vi "brat robotic.vi"() -> ()   [LabVIEW 2018]
uses:
  <vilib>/picture/3D Picture Control/Object/Create Object (name).vi
  <vilib>/picture/3D Picture Control/NI_3D Picture Control.lvlib
panel:
  in  "Angle":sgl(knob) scale=0.0..10.0
  in  "Axis":cluster{"X":sgl, "Y":sgl, "Z":sgl}
  in  "Y":sgl(slide)=-0.010994764 scale=-0.7..0.7
  in  "X":sgl(slide)=0.0074074073 scale=-0.7..0.7
  in  "stop":bool
  out "3D Picture":refnum<vi>(3d-picture)
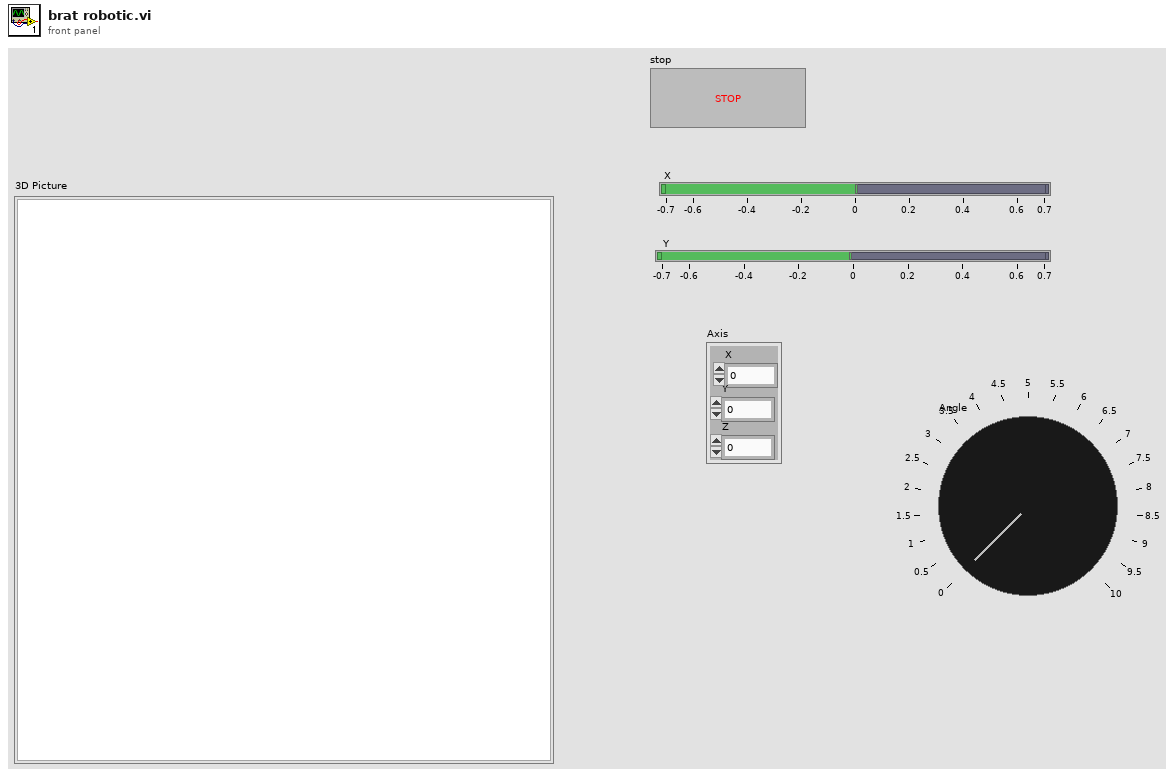
[diagram p1: front panel]
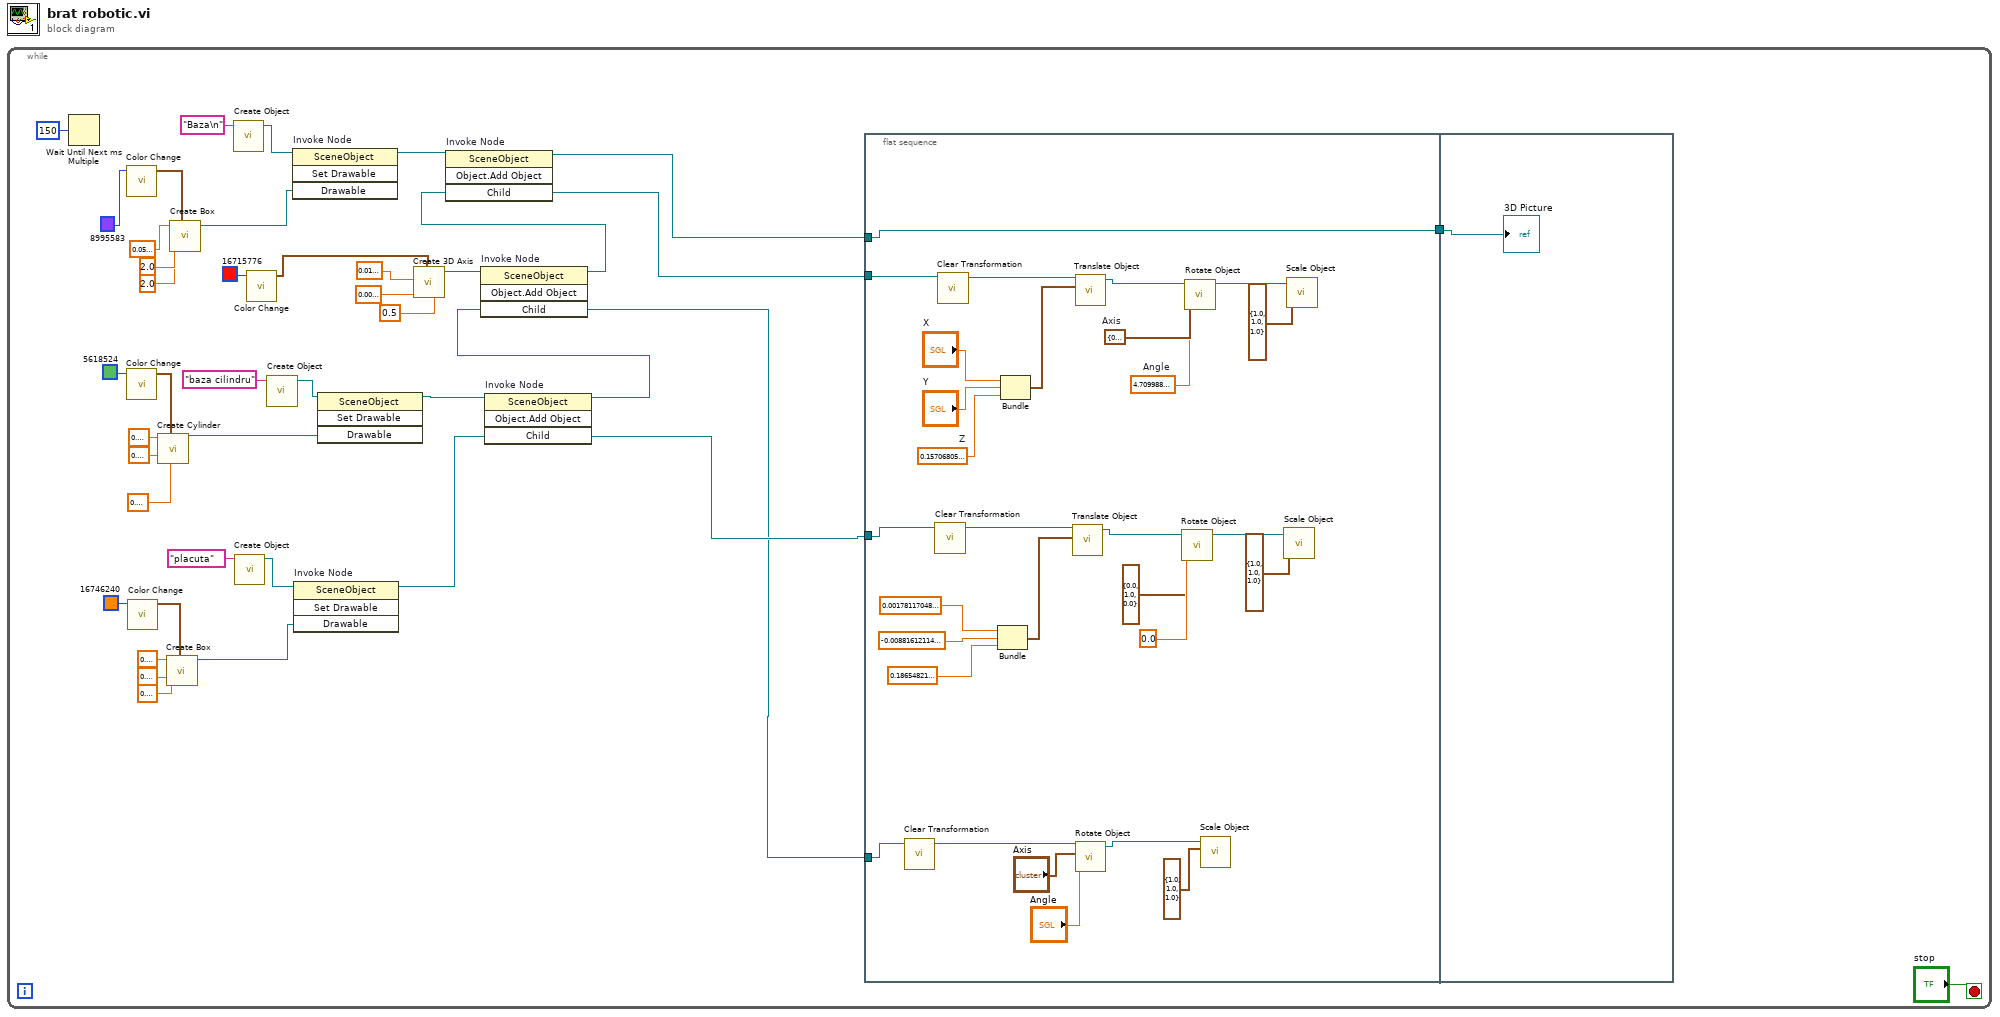
[diagram p0: block diagram]
diagram:
  n1 = while {
    stop <- "stop" stop-if-true
    n2 = Wait Until Next ms Multiple(millisecond multiple=u32 150) -> ()  [unwired: 1 out]
    n3 = call <vilib>:"Color Change.vi"("Color"=u32 8995583) -> ("RGBA"=w38:cluster{"R":sgl, "G":sgl, "B":sgl, "A":sgl})  [unwired: 10 in]
    n4 = call <vilib>:"Color Change.vi"("Color"=u32 5618524) -> ("RGBA"=w26:cluster{"R":sgl, "G":sgl, "B":sgl, "A":sgl})  [unwired: 10 in]
    n5 = call <vilib>:"Color Change.vi"("Color"=u32 16746240) -> ("RGBA"=w16:cluster{"R":sgl, "G":sgl, "B":sgl, "A":sgl})  [unwired: 10 in]
    n6 = call <vilib>:"Create Cylinder.vi"("Detail"=sgl 0.3, "Color"=w26, "Radius"=sgl 0.3, "Height"=sgl 0.3) -> ("New Cylinder Refnum"=w23:refnum<vi>)  [unwired: 6 in, 1 out]
    n7 = call <vilib>:"Create Box.vi"("Color"=w16, "Length Z"=sgl 0.1, "Length Y"=sgl 0.2, "Length X"=sgl 0.2) -> ("New Box Refnum"=w13:refnum<vi>)  [unwired: 6 in, 1 out]
    n8 = call <vilib>:"Create Box.vi"("Color"=w38, "Length Z"=sgl 2.0, "Length Y"=sgl 2.0, "Length X"=sgl 0.05) -> ("New Box Refnum"=w35:refnum<vi>)  [unwired: 6 in, 1 out]
    n9 = call-poly <vilib>:"Create Object.vi"("Name"="Baza\n") -> ("Scene:New Object"=w36:refnum<vi>)  [unwired: 9 in, 1 out]
    n10 = call-poly <vilib>:"Create Object.vi"("Name"="placuta") -> ("Scene:New Object"=w14:refnum<vi>)  [unwired: 9 in, 1 out]
    n11 = call <vilib>:"Color Change.vi"("Color"=u32 16715776) -> ("RGBA"=w6:cluster{"R":sgl, "G":sgl, "B":sgl, "A":sgl})  [unwired: 10 in]
    n12 = call-poly <vilib>:"Create Object.vi"("Name"="baza cilindru") -> ("Scene:New Object"=w24:refnum<vi>)  [unwired: 9 in, 1 out]
    n13 = invoke on="Invoke Node" class="SceneObject" method="Set Drawable"(reference=w36, "Drawable"=w35) -> (reference out=w32:refnum<vi>)  [unwired: 2 in, 3 out]
    n14 = invoke on="Invoke Node" class="SceneObject" method="Set Drawable"(reference=w14, "Drawable"=w13) -> (reference out=w11:refnum<vi>)  [unwired: 2 in, 3 out]
    n15 = invoke class="SceneObject" method="Set Drawable"(reference=w24, "Drawable"=w23) -> (reference out=w20:refnum<vi>)  [unwired: 2 in, 3 out]
    n16 = call <vilib>:"Create 3D Axis.vi"("Character Size"=sgl 0.5, "Color"=w6, "Radius"=sgl 0.01, "Length"=sgl 0.02) -> ("New Object Refnum"=w4:refnum<vi>)  [unwired: 6 in, 1 out]
    n17 = invoke on="Invoke Node" class="SceneObject" method="Object.Add Object"(reference=w20, "Child"=w11) -> (reference out=w3:refnum<vi>, "Child"=w10:refnum<vi>)  [unwired: 2 in, 2 out]
    n18 = invoke on="Invoke Node" class="SceneObject" method="Object.Add Object"(reference=w4, "Child"=w3) -> (reference out=w2:refnum<vi>, "Child"=w1:refnum<vi>)  [unwired: 2 in, 2 out]
    n19 = invoke on="Invoke Node" class="SceneObject" method="Object.Add Object"(reference=w32, "Child"=w2) -> (reference out=w31:refnum<vi>, "Child"=w22:refnum<vi>)  [unwired: 2 in, 2 out]
    n20 = flat-sequence {
      tunnel: w31 -> [w71]
      tunnel: w22 -> [w70]
      tunnel: [w71] -> w21
      tunnel: w10 -> [w49]
      tunnel: w1 -> [w48]
      tunnel: w21 -> [w72]
      frame #0 {
        w61 = sgl 0.15706806  # Z
        w65 = cluster{"X":sgl, "Y":sgl, "Z":sgl} {"X"=0.0, "Y"=1.0, "Z"=0.0}  # Axis
        w64 = sgl 4.709988  # Angle
        n21 = call <vilib>:"Clear Transformation.vi"("Object Refnum In"=w48) -> ("Object Refnum Out"=w47:refnum<vi>)  [unwired: 9 in, 1 out]
        n22 = call <vilib>:"Clear Transformation.vi"("Object Refnum In"=w49) -> ("Object Refnum Out"=w50:refnum<vi>)  [unwired: 9 in, 1 out]
        n23 = call <vilib>:"Clear Transformation.vi"("Object Refnum In"=w70) -> ("Object Refnum Out"=w69:refnum<vi>)  [unwired: 9 in, 1 out]
        n24 = Bundle("X 2"=sgl 0.0017811705, "Y 2"=sgl -0.008816121, "Z"=sgl 0.18654822) -> (w59:cluster{"X 2":sgl, "Y 2":sgl, "Z":sgl})  [unwired: 1 in]
        n25 = Bundle("X"="X", "Y"="Y", "Z"=w61) -> (w60:cluster{"X":sgl, "Y":sgl, "Z":sgl})  [unwired: 1 in]
        n26 = call <vilib>:"Translate Object.vi"("Translation"=w59, "Scene.Object In"=w50) -> ("Scene.Object Out"=w51:refnum<vi>)  [unwired: 8 in, 1 out]
        n27 = call <vilib>:"Translate Object.vi"("Translation"=w60, "Scene.Object In"=w69) -> ("Scene.Object Out"=w68:refnum<vi>)  [unwired: 8 in, 1 out]
        n28 = call <vilib>:"Rotate Object.vi"("Angle"="Angle", "Axis"="Axis", "Scene.Object In"=w47) -> ("Scene.Object Out"=w46:refnum<vi>)  [unwired: 7 in, 1 out]
        n29 = call <vilib>:"Rotate Object.vi"("Angle"=sgl 0.0, "Axis"=cluster{"X":sgl, "Y":sgl, "Z":sgl} {"X"=0.0, "Y"=1.0, "Z"=0.0}, "Scene.Object In"=w51) -> ("Scene.Object Out"=w52:refnum<vi>)  [unwired: 7 in, 1 out]
        n30 = call <vilib>:"Rotate Object.vi"("Angle"=w64, "Axis"=w65, "Scene.Object In"=w68) -> ("Scene.Object Out"=w67:refnum<vi>)  [unwired: 7 in, 1 out]
        n31 = call <vilib>:"Scale Object.vi"("Scale"=cluster{"X":sgl, "Y":sgl, "Z":sgl} {"X"=1.0, "Y"=1.0, "Z"=1.0}, "Scene.Object In"=w46) -> ()  [unwired: 8 in, 2 out]
        n32 = call <vilib>:"Scale Object.vi"("Scale"=cluster{"X":sgl, "Y":sgl, "Z":sgl} {"X"=1.0, "Y"=1.0, "Z"=1.0}, "Scene.Object In"=w52) -> ()  [unwired: 8 in, 2 out]
        n33 = call <vilib>:"Scale Object.vi"("Scale"=cluster{"X":sgl, "Y":sgl, "Z":sgl} {"X"=1.0, "Y"=1.0, "Z"=1.0}, "Scene.Object In"=w67) -> ()  [unwired: 8 in, 2 out]
      }
      frame #1 {
        "3D Picture" <- w72
      }
    }
  }
